vi "Write Read Scan to File.vi"(6 "Write":bool, 8 "error in":errorcluster, 9 "Tree Map in":T1, 11 "Path":path) -> (0 "error out":errorcluster, 1 "Tree Map Out":T1, 2 "Continue?":bool)   [LabVIEW 2019, in "Panther Dashboard.lvlib"]
uses:
  Panther Dashboard.lvlib
  <vilib>/National Instruments/Tree Map/Tree Map Data.ctl
  <vilib>/National Instruments/Tree Map/Tree Map.lvlib
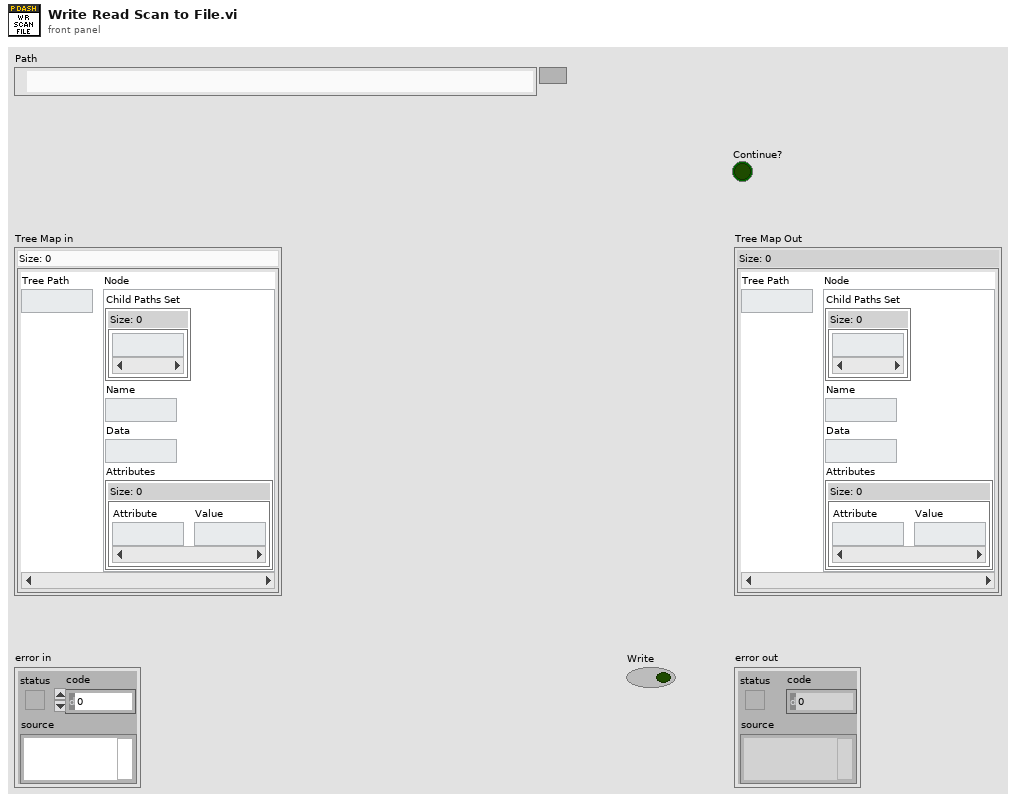
[diagram p1: front panel]
types:
  T1 = typedef "Tree Map.lvlib/Tree Map Data.ctl" = map{string, cluster{"Child Paths Set":set{string}, "Name":string, "Data":string, "Attributes":map{string, string}}}
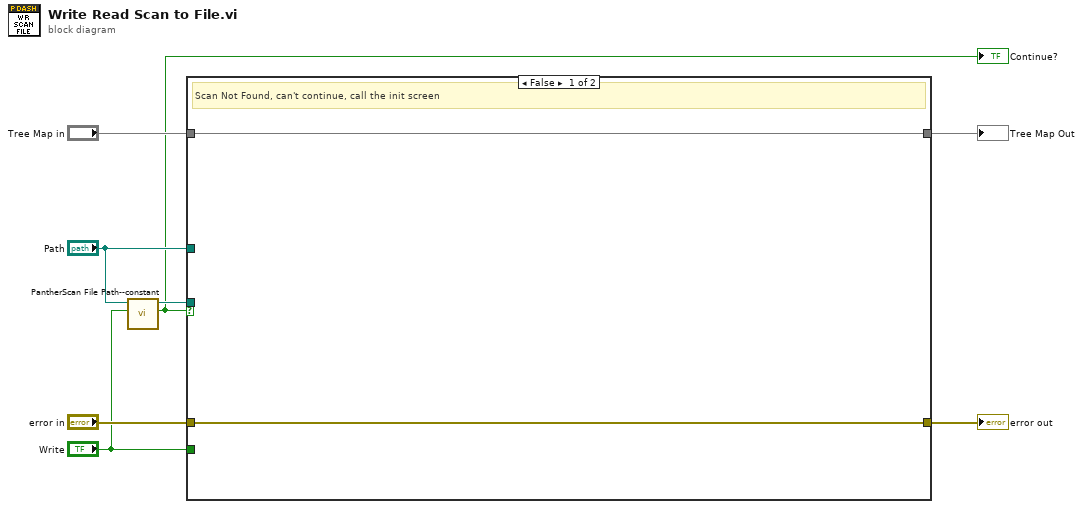
[diagram p0: block diagram]
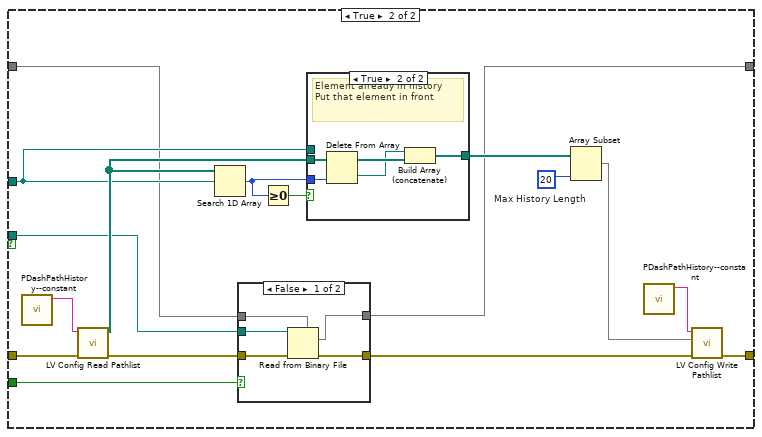
[diagram p2: hidden frame]
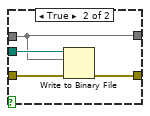
[diagram p3: hidden frame]
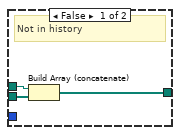
[diagram p4: hidden frame]
diagram:
  n1 = call "PantherScan File Path--constant.vi"("Write"="Write", "Path"="Path") -> ("Continue?"=w1:bool, "PantherScan file Path"=w6:path)  [unwired: 8 in]
  "Continue?" <- w1
  n2 = case shown="False" w1 {
    tunnel: [w10 w27] -> w8
    tunnel: "error in" -> [w10 w26]
    tunnel: w6 -> [_ w20]
    tunnel: "Path" -> [_ w16]
    tunnel: "Tree Map in" -> [w9 w13]
    tunnel: [w9 w12] -> w3
    tunnel: "Write" -> [_ w11]
    frame False {
      # "Scan Not Found, can't continue, call the init screen"
    }
    frame True {
      w17 = 20  # Max History Length
      n3 = call "PDashPathHistory--constant.vi"() -> ("PDashPathHistory"=w23:string)  [unwired: 11 in]
      n4 = call <resource>:"LV Config Read Pathlist.vi"("error in"=w26, "key"=w23) -> ("error out"=w25:errorcluster, "value"=w22:path[])  [unwired: 3 in, 1 out]
      n5 = Search 1D Array(1D array=w22, element=w16) -> (index of element=w14:i32)  [unwired: 1 in]
      n6 = case shown="False" w11 {
        tunnel: w25 -> [w32 w36]
        tunnel: [w31 w35] -> w24
        tunnel: w20 -> [w28 w34]
        tunnel: w13 -> [w30 w33]
        tunnel: [w29 w33] -> w12
        frame False {
          n7 = Read from Binary File(5:w30, 8:w32, 11:w28) -> (0:w31:errorcluster, 2:w29:T1)  [unwired: 3 in, 2 out]
        }
        frame True {
          n8 = Write to Binary File(file (use dialog)=w34, data=w33, error in=w36) -> (error out=w35:errorcluster)  [unwired: 3 in, 2 out]
        }
      }
      n9 = Greater Or Equal To 0?(x=w14) -> (x >= 0?=w21:bool)
      n10 = case shown="True" w21 {
        tunnel: w22 -> [w39 w44]
        tunnel: [w37 w42] -> w19
        tunnel: w16 -> [w38 _]
        tunnel: w14 -> [_ w43]
        frame False {
          # "Not in history"
          n11 = Build Array (concatenate)(w38, w39) -> (w37:path[])
        }
        frame True {
          # "Element already in history\nPut that element in front"
          n12 = Delete From Array(array=w44, index=w43) -> (deleted portion=w40:path, array with subset deleted=w41:path[])  [unwired: 1 in]
          n13 = Build Array (concatenate)(w40, w41) -> (w42:path[])
        }
      }
      n14 = Array Subset(array=w19, length=w17) -> (w18:path[])  [unwired: 1 in]
      n15 = call "PDashPathHistory--constant.vi"() -> ("PDashPathHistory"=w15:string)  [unwired: 11 in]
      n16 = call <resource>:"LV Config Write Pathlist.vi"("error in (no error)"=w24, "value"=w18, "key"=w15) -> ("error out"=w27:errorcluster)  [unwired: 4 in]
    }
  }
  "Tree Map Out" <- w3
  "error out" <- w8
